vi "Power On Dut.vi"(7 "measure call context in":refnum<class "Measure Call Context.lvclass">, 8 "error in":errorcluster, 11 "Power sequencing file path":path) -> (0 "error out":errorcluster, 5 "measure call context out":refnum<class "Measure Call Context.lvclass">)   [LabVIEW 2023]
uses:
  <vilib>/Plug-In SDKs/Measurements/Measure Call Context/Measure Call Context.lvclass
  <instrlib>/niDCPower/nidcpower.llb/niDCPower Source Mode.ctl
  <instrlib>/niDCPower/nidcpower.llb/niDCPower Output Function.ctl
  <instrlib>/niDCPower/nidcpower.llb/niDCPower gRPC Device Server.ctl
  NI gRPC Device Server - Action.ctl
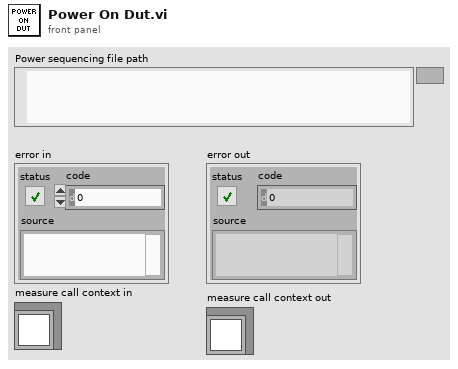
[diagram p1: front panel]
types:
  T1 = typedef "NI gRPC Device Server - Action.ctl" = enum16{"Start Server", "End Server"}
  T2 = typedef "DC Ins Initialize.ctl" = cluster{"Pin Name":string, "Resource Name":refnum<k15>, "Channel":string, "Voltage Range (V)":dbl, "Current Range (A)":dbl}
  T3 = typedef "DC Settings.ctl" = cluster{"Pin Name":string, "Resource Name":refnum<k15>, "Channel":string, "Power-up Seq":u32, "Power-up Voltage (V)":dbl, "Power-down Seq":u32, "Power-down Voltage (V)":dbl, "Current Limit (A)":dbl, "Wait Before Next (ms)":u32}
  T4 = typedef "niDCPower gRPC Device Server.ctl" = cluster{"session name":string, "address (localhost)":string, "port (31763)":u32}
  T5 = typedef "niDCPower Output Function.ctl" = i32
  T6 = typedef "niDCPower Source Mode.ctl" = i32
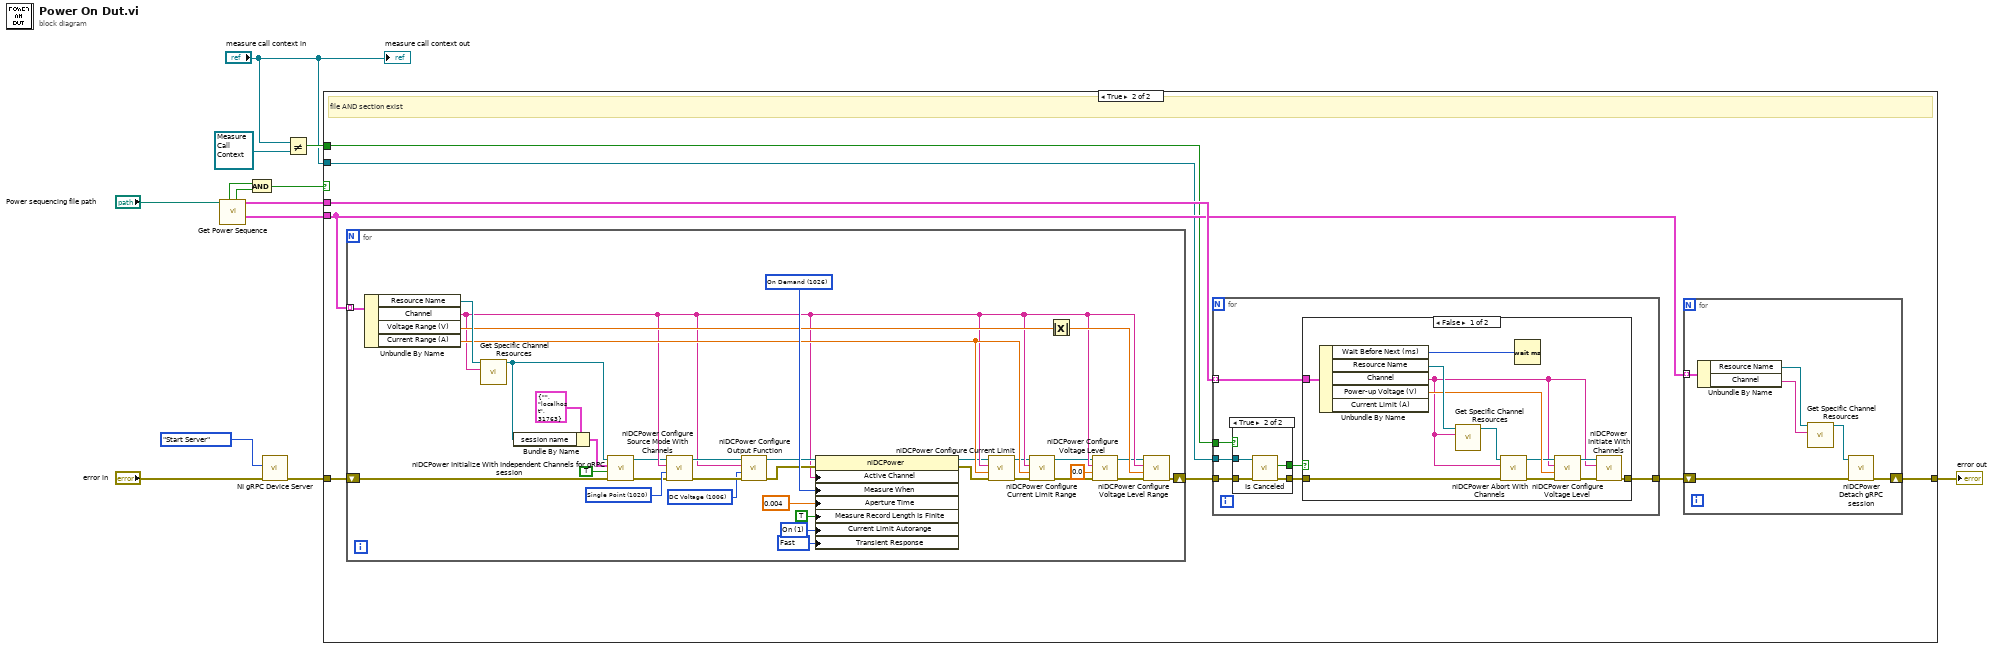
[diagram p0: block diagram]
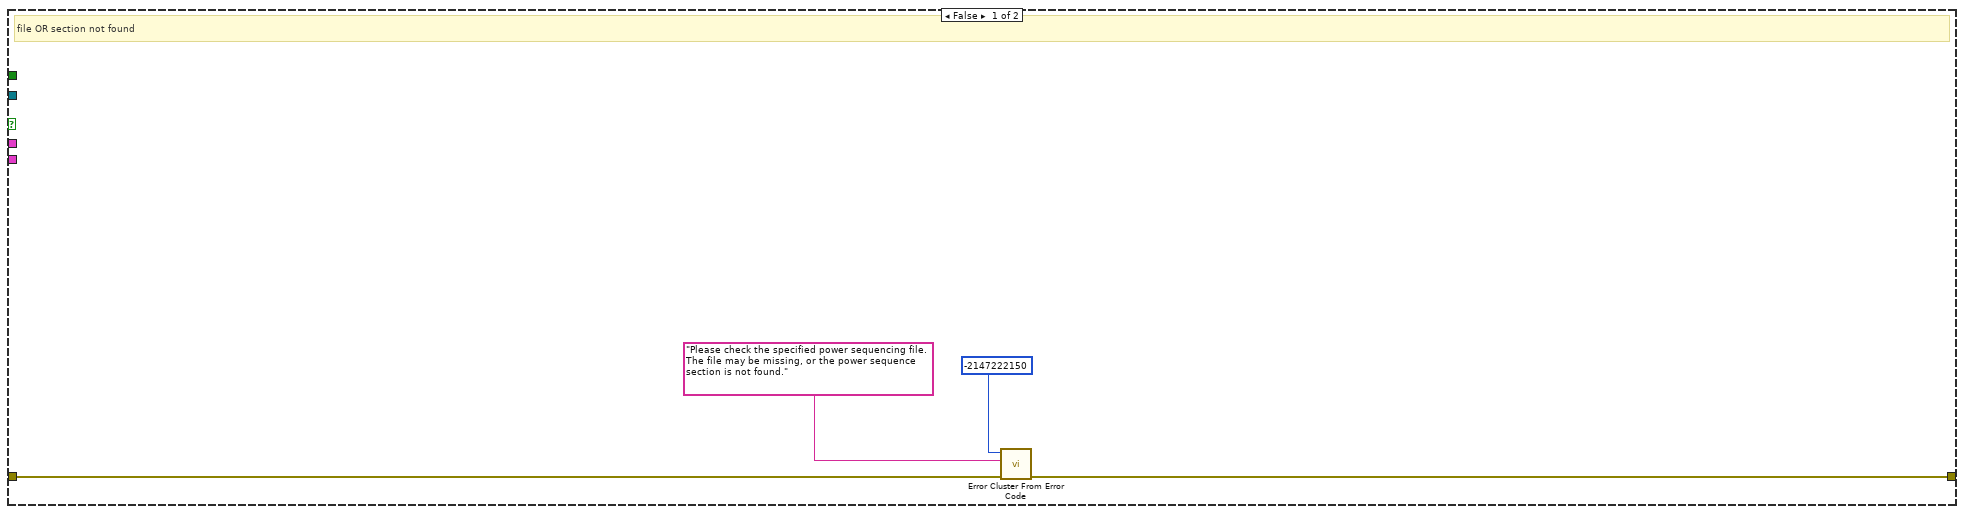
[diagram p2: hidden frame]
diagram:
  n1 = call "Get Power Sequence.vi"("File Path"="Power sequencing file path") -> ("SMUs to Initialize (not in order)"=w12:T2[], "Power up Seq"=w11:T3[], "File Exists?"=w7:bool, "Section Exists?"=w6:bool)  [unwired: 6 in, 1 out]
  n2 = And(x=w6, y=w7) -> (x .and. y?=w8:bool)
  n3 = call "NI gRPC Device Server.vi"("error in"="error in", "Action"=NI_gRPC_Device_Server_-_Action."Start Server") -> ("error out"=w5:errorcluster)  [unwired: 9 in]
  n4 = Not Equal?(x="measure call context in", y=refnum<class "Measure Call Context.lvclass"> refnum ("measure call context in")) -> (x != y?=w4:bool)
  n5 = case shown="True" w8 {
    tunnel: w12 -> [_ w20]
    tunnel: w11 -> [_ w25]
    tunnel: [w17 w21] -> w10
    tunnel: w5 -> [w16 w23]
    tunnel: "measure call context in" -> [_ w19]
    tunnel: w4 -> [_ w18]
    frame False {
      # "file OR section not found"
      n6 = call <vilib>:"Error Cluster From Error Code.vi"("error in (no error)"=w16, "error message (\"\")"="Please check the specified power sequencing file. The file may be missing, or the power sequence section is not found.", "error code (0)"=-2147222150) -> ("error out"=w17:errorcluster)  [unwired: 6 in]
    }
    frame True {
      # "file AND section exist"
      n7 = for {
        tunnel: w20 -> [w56] mode=indexing
        shift-right: [w40] -> w24
        shift-left: w23 -> [w58]
        w38 = 1039 items=["Slow"=1041, "Normal"=1038, "Fast"=1039, "Custom"=1042] ("Source:Transient Response")
        w39 = 1 items=["Off", "On"] ("Measurement:Autorange")
        w60 = 1026 items=["Automatically after Source Complete"=1025, "On Demand"=1026, "On Measure Trigger"=1027] ("Measurement:Advanced:Measure When")
        w61 = T5 1006 items=["DC Voltage"=1006, "DC Current"=1007, "Pulse Voltage"=1049, "Pulse Current"=1050] ("output function")
        w62 = T6 1020 items=["Single Point"=1020, "Sequence"=1021] ("source mode")
        n8 = Unbundle By Name(w56) -> ("Resource Name"=w65:refnum<k15>, "Channel"=w50:string, "Voltage Range (V)"=w53:dbl, "Current Range (A)"=w51:dbl)
        n9 = call "Get Specific Channel Resources.vi"("Channel"=w50, "Resource Name"=w65) -> ("Resource Name"=w32:refnum<k15>)  [unwired: 9 in]
        n10 = Bundle By Name(cluster=T4 {"session name"="", "address (localhost)"="localhost", "port (31763)"=31763} ("gRPC options"), "session name"=w32) -> (w33:T4)
        n11 = call <instrlib>:"niDCPower Initialize With Independent Channels for gRPC session.vi"("error in (no error)"=w58, "reset (false)"=TRUE, "gRPC options"=w33, "resource name"=w32) -> ("error out"=w35:errorcluster, "instrument handle out"=w36:refnum<k15>)  [unwired: 6 in]
        n12 = call <instrlib>:"niDCPower Configure Source Mode With Channels.vi"("error in (no error)"=w35, "source mode"=w62, "channel name"=w50, "instrument handle"=w36) -> ("error out"=w63:errorcluster, "instrument handle out"=w64:refnum<k15>)  [unwired: 6 in]
        n13 = call <instrlib>:"niDCPower Configure Output Function.vi"("error in (no error)"=w63, "output function"=w61, "channel name"=w50, "instrument handle"=w64) -> ("error out"=w54:errorcluster, "instrument handle out"=w55:refnum<k15>)  [unwired: 6 out]
        n14 = property class="niDCPower"(reference=w55, error in=w54, "Active Channel"=w50, "Measure When"=w60, "Aperture Time"=0.004 ("Measurement:Aperture Time"), "Measure Record Length Is Finite"=TRUE ("Measurement:Measure Record Length Is Finite"), "Current Limit Autorange"=w39, "Transient Response"=w38) -> (reference out=w48:refnum<k15>, error out=w47:errorcluster)
        n15 = call <instrlib>:"niDCPower Configure Current Limit.vi"("error in (no error)"=w47, "current limit"=w51, "channel name"=w50, "instrument handle"=w48) -> ("error out"=w45:errorcluster, "instrument handle out"=w46:refnum<k15>)  [unwired: 1 in, 5 out]
        n16 = call <instrlib>:"niDCPower Configure Current Limit Range.vi"("error in (no error)"=w45, "current limit range"=w51, "channel name"=w50, "instrument handle"=w46) -> ("error out"=w43:errorcluster, "instrument handle out"=w44:refnum<k15>)  [unwired: 6 out]
        n17 = Absolute Value(x=w53) -> (abs(x)=w52:dbl)
        n18 = call <instrlib>:"niDCPower Configure Voltage Level.vi"("error in (no error)"=w43, "voltage level"=0.0, "channel name"=w50, "instrument handle"=w44) -> ("error out"=w41:errorcluster, "instrument handle out"=w42:refnum<k15>)  [unwired: 6 in]
        n19 = call <instrlib>:"niDCPower Configure Voltage Level Range.vi"("error in (no error)"=w41, "voltage level range"=w52, "channel name"=w50, "instrument handle"=w42) -> ("error out"=w40:errorcluster)  [unwired: 7 out]
      }
      n20 = for {
        tunnel: w25 -> [w72] mode=indexing
        tunnel: w24 -> [w69]
        tunnel: [w71] -> w22
        tunnel: w19 -> [w67]
        tunnel: w18 -> [w66]
        n21 = case shown="True" w66 {
          tunnel: [_ w77] -> w70
          tunnel: w69 -> [w73 w76]
          tunnel: [w73 w75] -> w68
          tunnel: w67 -> [_ w74]
          frame False {
          }
          frame True {
            n22 = call <vilib>:"Is Canceled.vi"("error in"=w76, "measure call context in"=w74) -> ("error out"=w75:errorcluster, "is canceled?"=w77:bool)  [unwired: 7 in, 1 out]
          }
        }
        n23 = case shown="False" w70 {
          tunnel: w72 -> [w87 _]
          tunnel: w68 -> [w82 w90]
          tunnel: [w78 w90] -> w71
          frame False {
            n24 = Unbundle By Name(w87) -> ("Wait Before Next (ms)"=w88:u32, "Resource Name"=w89:refnum<k15>, "Channel"=w79:string, "Power-up Voltage (V)"=w84:dbl)  [unwired: 1 out]
            n25 = call "Get Specific Channel Resources.vi"("Channel"=w79, "Resource Name"=w89) -> ("Resource Name"=w86:refnum<k15>)  [unwired: 9 in]
            n26 = call <instrlib>:"niDCPower Abort With Channels.vi"("error in (no error)"=w82, "channel name"=w79, "instrument handle"=w86) -> ("error out"=w80:errorcluster, "instrument handle out"=w81:refnum<k15>)  [unwired: 7 in]
            n27 = Wait (ms)(milliseconds to wait=w88) -> ()  [unwired: 1 out]
            n28 = call <instrlib>:"niDCPower Configure Voltage Level.vi"("error in (no error)"=w80, "voltage level"=w84, "channel name"=w79, "instrument handle"=w81) -> ("error out"=w83:errorcluster, "instrument handle out"=w85:refnum<k15>)  [unwired: 6 in]
            n29 = call <instrlib>:"niDCPower Initiate With Channels.vi"("error in (no error)"=w83, "channel name"=w79, "instrument handle"=w85) -> ("error out"=w78:errorcluster)  [unwired: 7 in, 1 out]
          }
          frame True {
          }
        }
      }
      n30 = for {
        shift-right: [w30] -> w21
        shift-left: w22 -> [w31]
        tunnel: w20 -> [w29] mode=indexing
        n31 = Unbundle By Name(w29) -> ("Resource Name"=w27:refnum<k15>, "Channel"=w26:string)
        n32 = call "Get Specific Channel Resources.vi"("Channel"=w26, "Resource Name"=w27) -> ("Resource Name"=w28:refnum<k15>)  [unwired: 9 in]
        n33 = call <instrlib>:"niDCPower Detach gRPC session.vi"("error in (no error)"=w31, "instrument handle"=w28) -> ("error out"=w30:errorcluster)  [unwired: 9 in]
      }
    }
  }
  "error out" <- w10
  "measure call context out" <- "measure call context in"
